vi "fpga_Equal 1.vi"(11 "data in 32.0":fxp<+,32,0>=0.9999999997671694) -> (3 "=1?":bool)   [LabVIEW 2012, in "NI_EP_Protection_FPGA.lvlib"]
uses:
  <vilib>/addons/Electrical Power/Protection/NI_EP_Protection_FPGA.lvlib
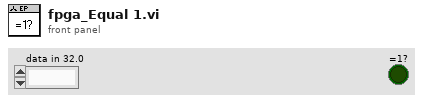
[diagram p1: front panel]
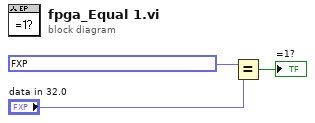
[diagram p0: block diagram]
diagram:
  n1 = Equal?(x=fxp<+,32,0> 0.9999999997671694 ("x+y"), y="data in 32.0") -> (x = y?=→"=1?":bool)
